vi "LB_IndexArray.vi"(11 "error in (no error)":errorcluster) -> (15 "error out":errorcluster)   [LabVIEW 2016, in "DronaTest.lvlib"]
uses:
  DronaTest.lvlib
  APIs/Stimulus/ControlValue/SetValueAuto.vi
  APIs/Stimulus/ControlValue/Controls/Listbox/SetValueByArrayIndex.vi
  APIs/Assert/AssertControlValue/Equal.vi
  <vilib>/addons/_JKI Toolkits/Caraya/classes/Assert/Assert Error.vi
  APIs/Stimulus/VI/CloseVI.vi
  <vilib>/addons/_JKI Toolkits/Caraya/classes/Test/Test.lvclass
  Drona.lvlib
  <vilib>/SLL Toolkit/SLL Debug/SLL Debug.lvlib
  APIs/Stimulus/ControlValue/ControlValue.lvlib
  APIs/Stimulus/ControlValue/Controls/Listbox/StimulusListbox.lvlib
  APIs/Assert/AssertControlValue/AssertControlValue.lvlib
  <vilib>/addons/_JKI Toolkits/Caraya/classes/Assert/Assert.lvclass
  APIs/Stimulus/VI/VI.lvlib
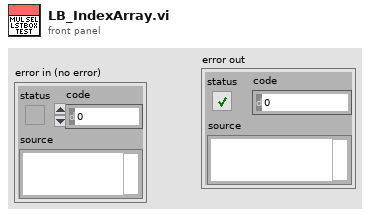
[diagram p1: front panel]
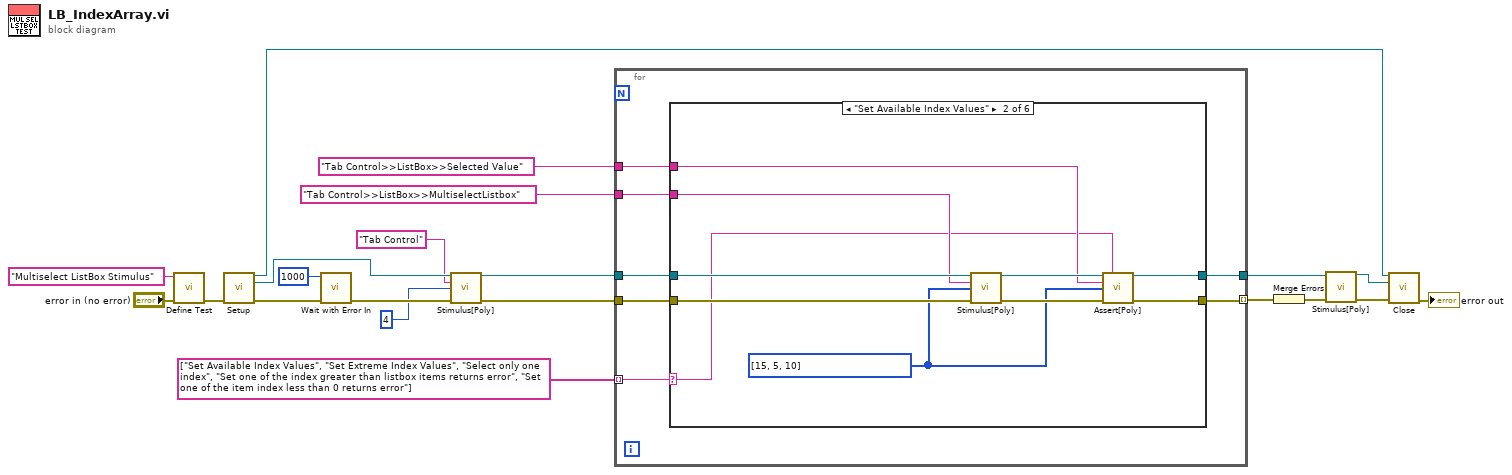
[diagram p0: block diagram]
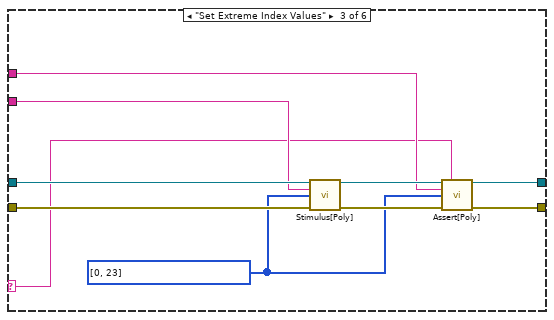
[diagram p3: hidden frame]
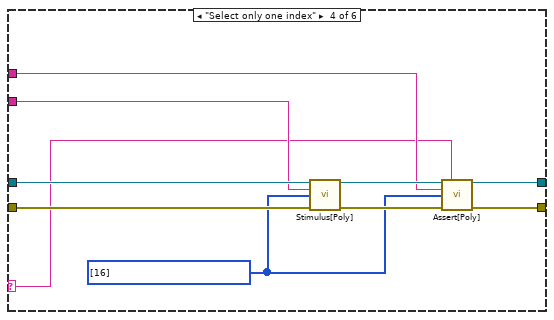
[diagram p4: hidden frame]
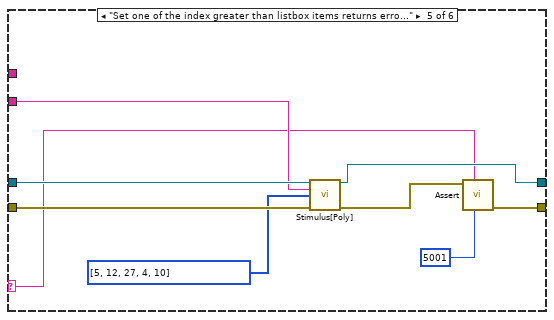
[diagram p5: hidden frame]
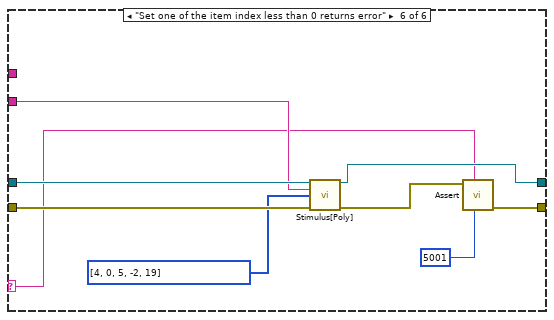
[diagram p6: hidden frame]
diagram:
  n1 = call <vilib>:"Define Test.vi"("error in (no error)"="error in (no error)", "Label (VI Title)"="Multiselect ListBox Stimulus") -> ("error out"=w20:errorcluster)  [unwired: 9 in]
  n2 = call "Setup.vi"("error in"=w20) -> ("Application Ref"=w5:refnum<vi>, "VI Reference Out"=w14:refnum<vi>, "error out"=w19:errorcluster)  [unwired: 12 in]
  n3 = call <vilib>:"Wait with Error In.vi"("error in (no error)"=w19, "milliseconds to wait"=u32 1000) -> ("error out"=w16:errorcluster)  [unwired: 9 in]
  n4 = call-poly "Stimulus[Poly].vi"("VI Reference In"=w14, "Control Path"="Tab Control", "Value (Signaling)"=4, "error in"=w16) -> ("VI Reference Out"=w10:refnum<vi>, "error out"=w15:errorcluster)  [unwired: 10 in]
  n5 = for {
    tunnel: w15 -> [w28]
    tunnel: w10 -> [w27]
    tunnel: "Tab Control>>ListBox>>MultiselectListbox" ("Control Path") -> [w26]
    tunnel: "Tab Control>>ListBox>>Selected Value" ("Control Path") -> [w25]
    tunnel: [w24] -> w2 mode=indexing
    tunnel: [w23] -> w4
    tunnel: string[] ["Set Available Index Values", "Set Extreme Index Values", "Select only one index", "Set one of the index greater than listbox items returns error", "Set one of the item index less than 0 returns error"] -> [w22] mode=indexing
    n6 = case shown="\"Set Available Index Values\"" w22 {
      selector: w22 -> [_ w31 w41 w51 w63 w72]
      tunnel: w28 -> [w30 w40 w50 w60 w69 w78]
      tunnel: w27 -> [w29 w39 w49 w59 w68 w77]
      tunnel: w26 -> [_ w38 w48 w58 w67 w76]
      tunnel: w25 -> [_ w35 w45 w55 _ _]
      tunnel: [w30 w33 w43 w53 w65 w74] -> w24
      tunnel: [w29 w32 w42 w52 w64 w73] -> w23
      frame Default {
      }
      frame "Set Available Index Values" {
        w34 = i32[] [15, 5, 10] ("Index Array")
        n7 = call-poly "Stimulus[Poly].vi"("VI Reference In"=w39, "Control Path"=w38, "Index Array"=w34, "Error In"=w40) -> ("VI Reference Out"=w36:refnum<vi>, "Error Out"=w37:errorcluster)  [unwired: 10 in]
        n8 = call-poly "Assert[Poly].vi"("VI Reference In"=w36, "Test Label"=w31, "Control Path"=w35, "Control Value"=w34, "Error In"=w37) -> ("VI Reference Out"=w32:refnum<vi>, "Error Out"=w33:errorcluster)  [unwired: 8 in, 1 out]
      }
      frame "Set Extreme Index Values" {
        w44 = i32[] [0, 23] ("Index Array")
        n9 = call-poly "Stimulus[Poly].vi"("VI Reference In"=w49, "Control Path"=w48, "Index Array"=w44, "Error In"=w50) -> ("VI Reference Out"=w46:refnum<vi>, "Error Out"=w47:errorcluster)  [unwired: 10 in]
        n10 = call-poly "Assert[Poly].vi"("VI Reference In"=w46, "Test Label"=w41, "Control Path"=w45, "Control Value"=w44, "Error In"=w47) -> ("VI Reference Out"=w42:refnum<vi>, "Error Out"=w43:errorcluster)  [unwired: 8 in, 1 out]
      }
      frame "Select only one index" {
        w54 = i32[] [16] ("Index Array")
        n11 = call-poly "Stimulus[Poly].vi"("VI Reference In"=w59, "Control Path"=w58, "Index Array"=w54, "Error In"=w60) -> ("VI Reference Out"=w56:refnum<vi>, "Error Out"=w57:errorcluster)  [unwired: 10 in]
        n12 = call-poly "Assert[Poly].vi"("VI Reference In"=w56, "Test Label"=w51, "Control Path"=w55, "Control Value"=w54, "Error In"=w57) -> ("VI Reference Out"=w52:refnum<vi>, "Error Out"=w53:errorcluster)  [unwired: 8 in, 1 out]
      }
      frame "Set one of the index greater than listbox items returns error" {
        n13 = call-poly "Stimulus[Poly].vi"("VI Reference In"=w68, "Control Path"=w67, "Index Array"=i32[] [5, 12, 27, 4, 10], "Error In"=w69) -> ("VI Reference Out"=w64:refnum<vi>, "Error Out"=w62:errorcluster)  [unwired: 10 in]
        n14 = call-poly <vilib>:"Assert.vi"("error code (1)"=5001, "Label"=w63, "Error?"=w62) -> ("error out"=w65:errorcluster)  [unwired: 8 in]
      }
      frame "Set one of the item index less than 0 returns error" {
        n15 = call-poly "Stimulus[Poly].vi"("VI Reference In"=w77, "Control Path"=w76, "Index Array"=i32[] [4, 0, 5, -2, 19], "Error In"=w78) -> ("VI Reference Out"=w73:refnum<vi>, "Error Out"=w71:errorcluster)  [unwired: 10 in]
        n16 = call-poly <vilib>:"Assert.vi"("error code (1)"=5001, "Label"=w72, "Error?"=w71) -> ("error out"=w74:errorcluster)  [unwired: 8 in]
      }
    }
  }
  n17 = Merge Errors(w2) -> (w3:errorcluster)
  n18 = call-poly "Stimulus[Poly].vi"("VI Reference In"=w4, "error in"=w3) -> ("VI Reference Out"=w7:refnum<vi>, "error out"=w6:errorcluster)  [unwired: 12 in]
  n19 = call "Close.vi"("Application Ref"=w5, "VI Reference"=w7, "error in"=w6) -> ("error out"=→"error out":errorcluster)  [unwired: 12 in]
